vi "Day 20 - Grove Positioning System.vi"() -> ()   [LabVIEW 2020, in "AoC 2022.lvlib"]
uses:
  AoC 2022.lvlib
  cf577a35-b93e-465b-a919-1c578a9c2c2d.vi
  f8efda8d-d27f-445e-9869-31da807afce3.vi
  26d2b5a9-47bc-4e61-9de5-45b045caeb60.vi
  fdc7296d-8aeb-47d2-a305-2f6f5ee265d9.vi
panel:
  out "Puzzle Part 2 Answer":i64
  out "Puzzle Answer":i64
  in  "Puzzle Input":string="1\n2\n-3\n3\n-2\n0\n4"
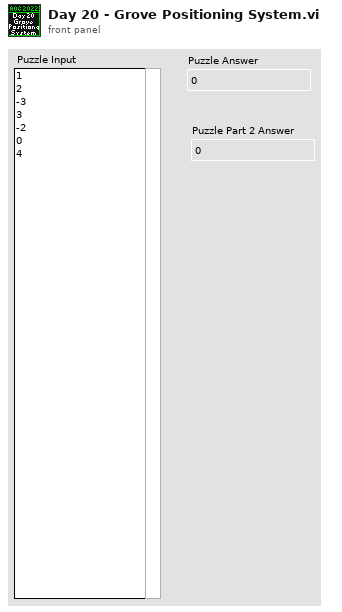
[diagram p1: front panel]
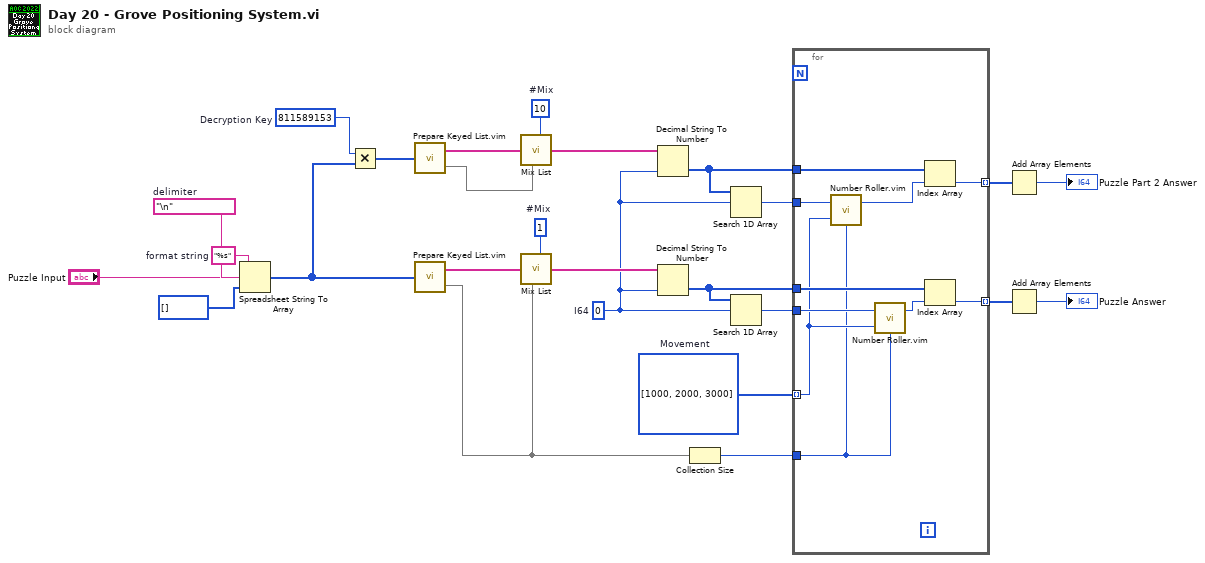
[diagram p0: block diagram]
diagram:
  w9 = 10  # #Mix
  w13 = 1  # #Mix
  w4 = i64 0  # I64
  w16 = i64 811589153  # Decryption Key
  w20 = i32[] [1000, 2000, 3000]  # Movement
  w25 = "%s"  # format string
  w26 = "\n"  # delimiter
  n1 = Spreadsheet String To Array(delimiter (Tab)=w26, format string=w25, spreadsheet string="Puzzle Input", array type (2D Dbl)=i64[] []) -> (array=w11:i64[])
  n2 = Multiply(x=w16, y=w11) -> (x*y=w10:i64[])
  n3 = call "Prepare Keyed List.vim"("List in"=w10) -> ("Keyed List"=w8:string[], "List Order"=w7:map{i32, string})
  n4 = call "Prepare Keyed List.vim"("List in"=w11) -> ("Keyed List"=w15:string[], "List Order"=w14:map{i32, string})
  n5 = call "Mix List.vi"("List in"=w8, "List Order"=w7, "#Mix"=w9) -> ("List out"=w6:string[])
  n6 = call "Mix List.vi"("List in"=w15, "List Order"=w14, "#Mix"=w13) -> ("List out"=w12:string[])
  n7 = Decimal String To Number(string=w6, default (0L)=w4) -> (number=w5:i64[])  [unwired: 1 in, 1 out]
  n8 = Decimal String To Number(string=w12, default (0L)=w4) -> (number=w21:i64[])  [unwired: 1 in, 1 out]
  n9 = Collection Size(1:w14) -> (0:w17:i32)
  n10 = Search 1D Array(1D array=w5, element=w4) -> (index of element=w3:i32)  [unwired: 1 in]
  n11 = Search 1D Array(1D array=w21, element=w4) -> (index of element=w22:i32)  [unwired: 1 in]
  n12 = for {
    tunnel: w22 -> [w34]
    tunnel: w20 -> [w29] mode=indexing
    tunnel: w17 -> [w28]
    tunnel: w21 -> [w35]
    tunnel: [w36] -> w18 mode=indexing
    tunnel: w5 -> [w31]
    tunnel: w3 -> [w30]
    tunnel: [w27] -> w2 mode=indexing
    n13 = call "Number Roller.vim"("Current Value"=w30, "Max Range"=w28, "Movement"=w29) -> ("Next Value"=w32:i32)  [unwired: 1 out]
    n14 = call "Number Roller.vim"("Current Value"=w34, "Max Range"=w28, "Movement"=w29) -> ("Next Value"=w33:i32)  [unwired: 1 out]
    n15 = Index Array(array=w31, index=w32) -> (element=w27:i64)
    n16 = Index Array(array=w35, index=w33) -> (element=w36:i64)
  }
  n17 = Add Array Elements(numeric array=w2) -> (sum=→"Puzzle Part 2 Answer":i64)
  n18 = Add Array Elements(numeric array=w18) -> (sum=→"Puzzle Answer":i64)
